vi "Task 1.vi"() -> ()   [LabVIEW 2025]
doc: "Generating random numbers and inserting values to multi column listbox using event strustures"
uses:
  <vilib>/numeric/Random Number (Range) U64.vi
  <vilib>/numeric/sub_Random U32.vi
panel:
  in  "?":bool
  in  "stop":bool
  out "Output":i32(listbox)
  # "Generating random numbers and inserting values to multi column listbox using event strustures"
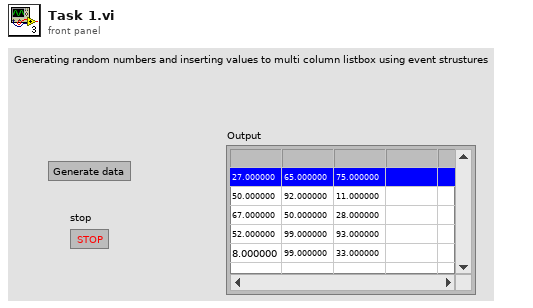
[diagram p1: front panel]
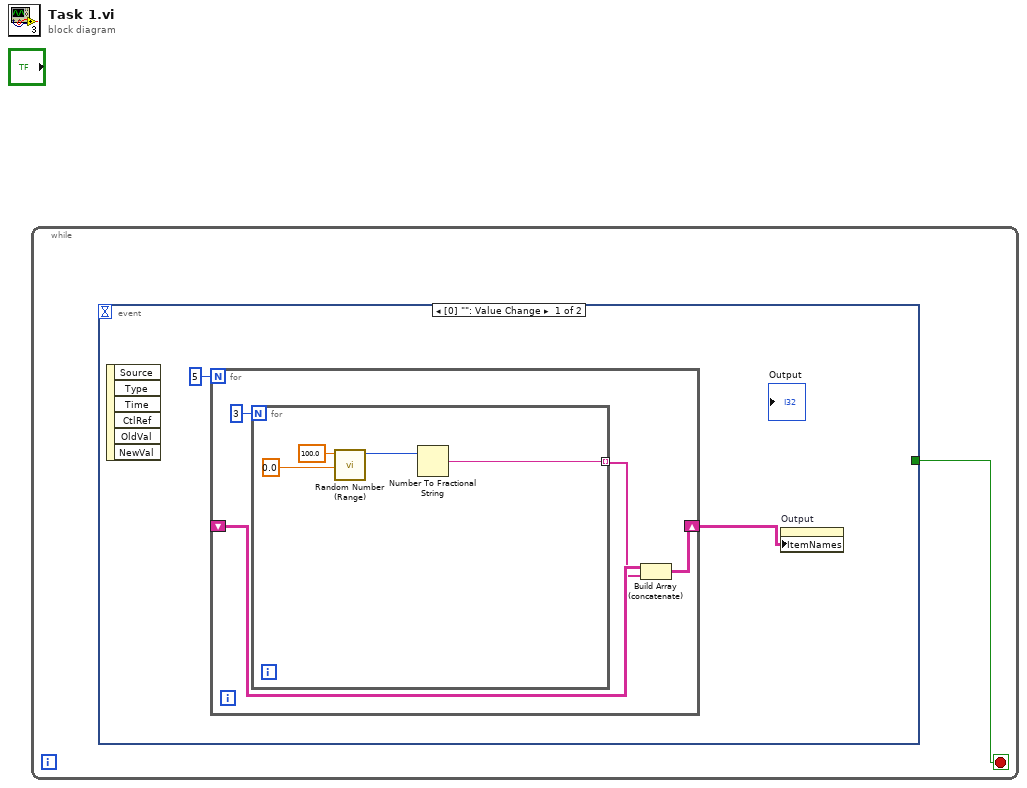
[diagram p0: block diagram]
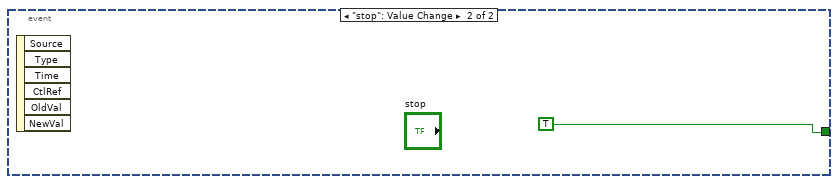
[diagram p2: hidden frame]
diagram:
  n1 = while {
    stop <- w1 stop-if-true
    n2 = event shown="[0] \"\": Value Change" {
      selector: _ -> [_ _]
      dyn-events: _ -> [_ _]
      timeout: _ -> [_ _]
      tunnel: [_ TRUE] -> w1
      event Value Change {
        n3 = event-data() -> ()  [unwired: 1 in, 6 out]
        n4 = for {
          N: 5 -> [_]
          shift-right: [w5] -> w2
          shift-left: _ -> [w6]
          n5 = for {
            N: 3 -> [_]
            tunnel: [w8] -> w4 mode=indexing
            n6 = call-poly <vilib>:"Random Number (Range).vi"("lower bound (0)"=0.0, "upper bound (100)"=100.0) -> ("number"=w9:u64)  [unwired: 9 in]
            n7 = Number To Fractional String(number=w9) -> (F-format string=w8:string)  [unwired: 3 in]
          }
          n8 = Build Array (concatenate)(w6, w4) -> (w5:string[][])
        }
        n9 = property on="Output" class="MCListbox (strict)"("ItemNames"=w2) -> ()  [unwired: 2 in, 2 out]
      }
      event "stop": Value Change {
        n10 = event-data() -> ()  [unwired: 1 in, 6 out]
      }
    }
  }
